vi "StringValueTest.vi"(4 "String":string="..\\..\\Models\\BusSupport") -> ()   [LabVIEW 2012]
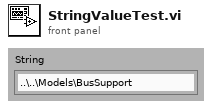
[diagram p1: front panel]
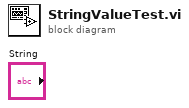
[diagram p0: block diagram]
diagram:
